vi "LcWebView_BubblePlot_Example.vi"() -> ()   [LabVIEW 2018, in "LcWebView.lvclass"]
doc: "Inject javascript arguments"
uses:
  LcWebView.lvclass
  plots/ctrls/PlotType.ctl
  plots/ctrls/GenericPlotOption.ctl
  plots/ctrls/LegendPosition.ctl
  C:/Users/ziggz/OneDrive/Documents/GitHub/LcWebView2/LcWebView/data/Microsoft.Web.WebView2.WinForms.dll
  Documents/GitHub/LcWebView2/LcWebView/data/Microsoft.Web.WebView2.WinForms.dll
panel:
  out "BrowserProcessId":u32
  out "Status Message":string
  in  "stop":bool
  in  "Web":refnum<k24>(container)
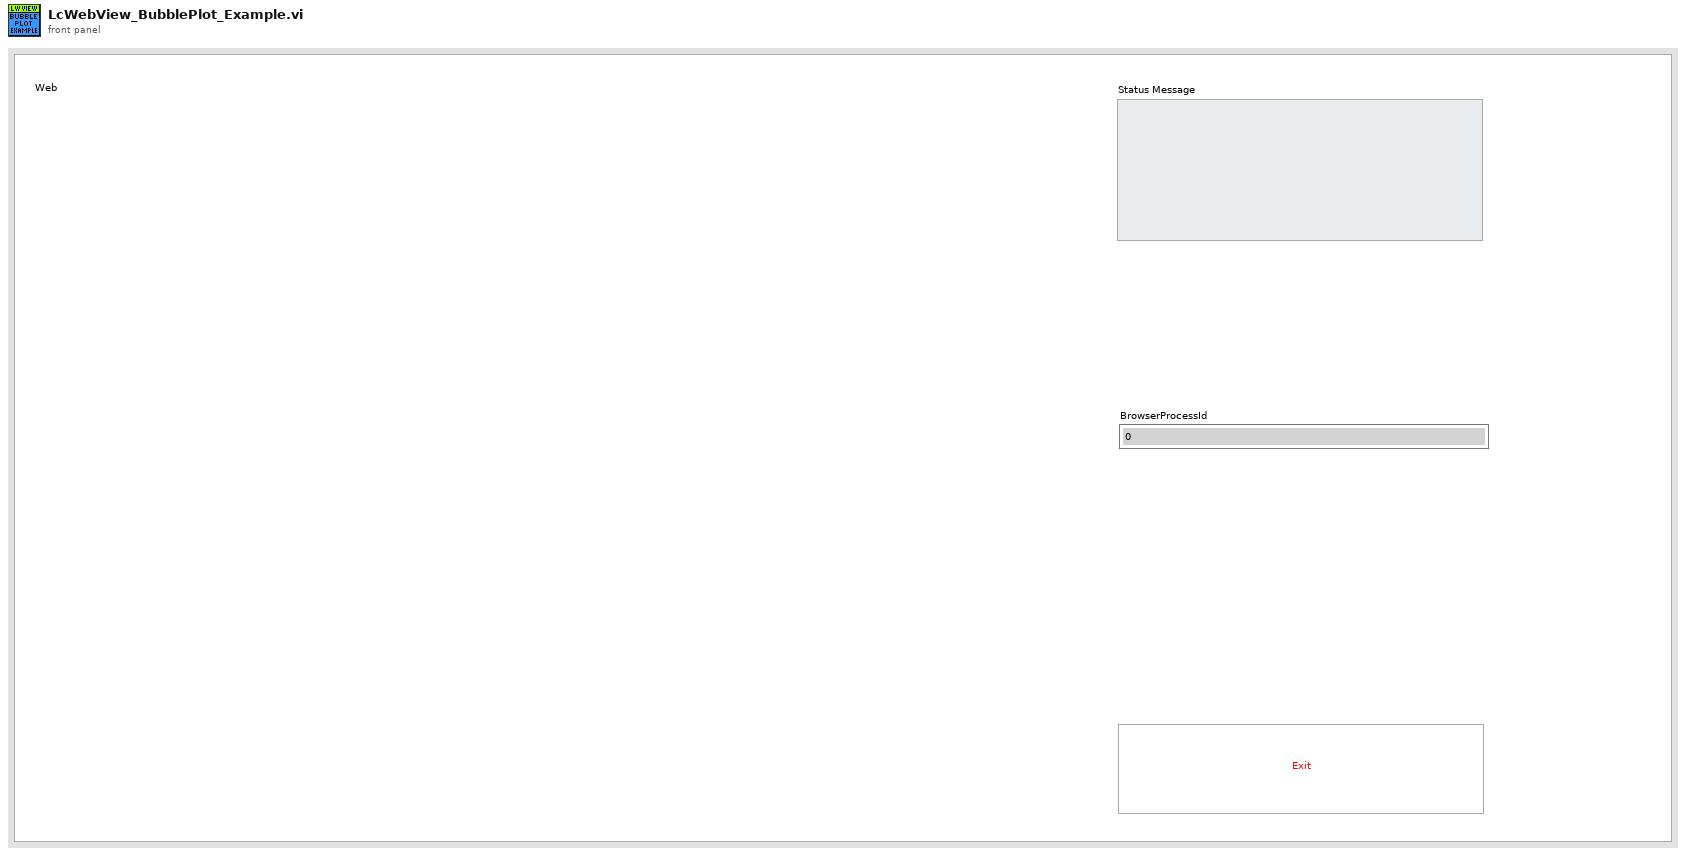
[diagram p1: front panel]
types:
  T1 = typedef "LcWebView.lvclass/GenericPlotOption.ctl" = cluster{"GraphTitle":string, "LegendDisplay":bool, "LegendPosition":T2}
  T2 = typedef "LcWebView.lvclass/LegendPosition.ctl" = enum16{"top", "right", "left", "bottom"}
  T3 = typedef "LcWebView.lvclass/PlotType.ctl" = enum16{"bar", "line", "pie", "doughnut", "scatter", "radar", "bubble", "polarArea"}
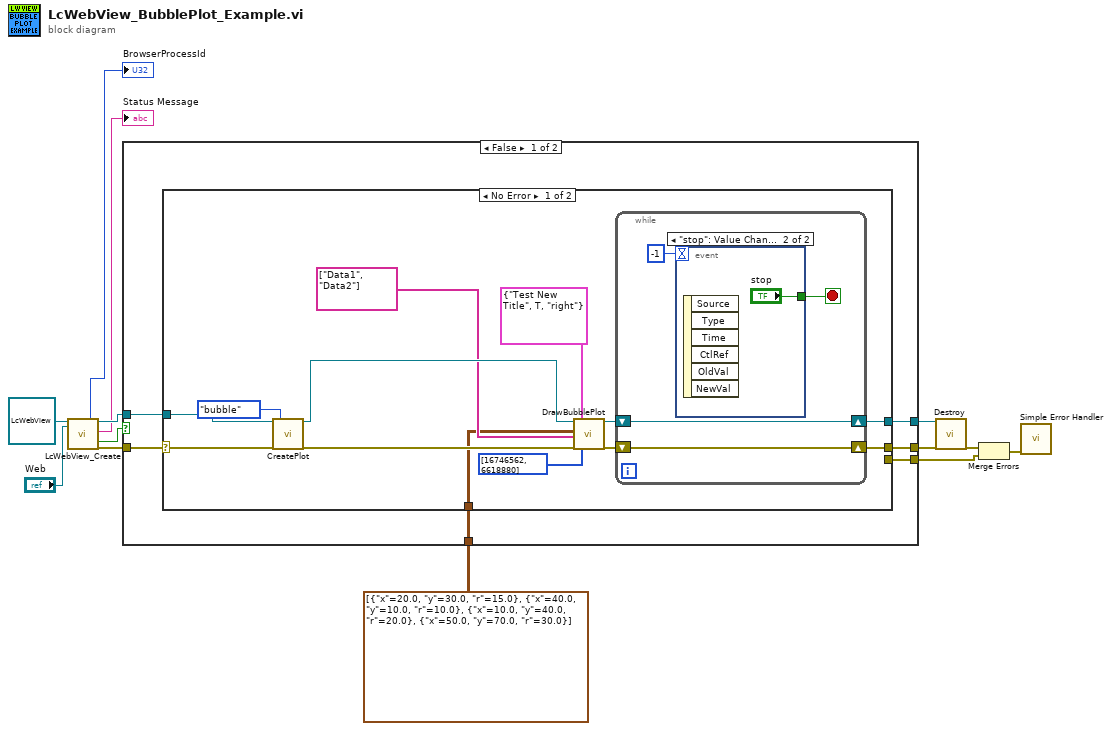
[diagram p0: block diagram]
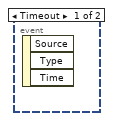
[diagram p2: hidden frame]
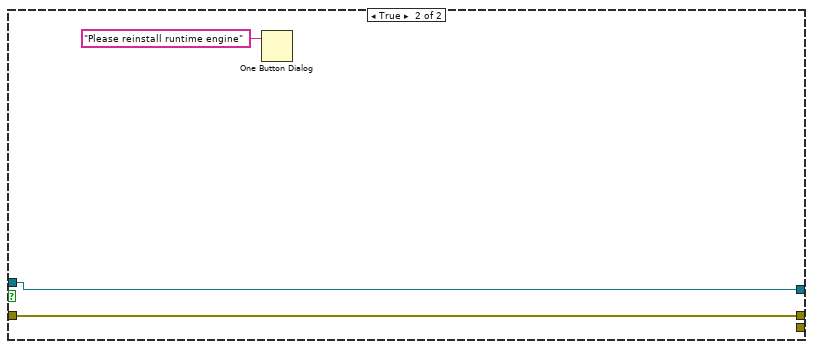
[diagram p4: hidden frame]
diagram:
  n1 = call "LcWebView_Create.vi"("reference in"=refnum<class "LcWebView.lvclass"> refnum, "Webview container"="Web") -> ("BrowserProcessId"=→"BrowserProcessId":u32, "reference out"=w11:refnum<class "LcWebView.lvclass">, "Status Message"=→"Status Message":string, "Reinstall Runtime"=w4:bool, "Error Out"=w10:errorcluster)  [unwired: 10 in, 3 out]
  n2 = case shown="False" w4 {
    tunnel: w11 -> [w19 w42]
    tunnel: w10 -> [w18 w41]
    tunnel: [w17 w42] -> w9
    tunnel: [w15 w41] -> w8
    tunnel: [w16 _] -> w5
    tunnel: cluster{"x":dbl, "y":dbl, "r":dbl}[][] [[{"x"=20.0, "y"=30.0, "r"=15.0}, {"x"=40.0, "y"=10.0, "r"=10.0}], [{"x"=10.0, "y"=40.0, "r"=20.0}, {"x"=50.0, "y"=70.0, "r"=30.0}]] ("BubblePlot.Dataset") -> [w14 _]
    frame False {
      n3 = case shown="No Error" w18 {
        selector: w18 -> [w30 w38]
        tunnel: w19 -> [w31 w39]
        tunnel: [w29 w39] -> w17
        tunnel: [w32 _] -> w15
        tunnel: [_ w38] -> w16
        tunnel: w14 -> [w20 _]
        frame No Error {
          n4 = call-dynamic "CreatePlot.vi"("reference in"=w31, "Error In"=w30, "PlotType"=PlotType."bubble") -> ("reference out"=w28:refnum<class "LcWebView.lvclass">, "Error Out"=w25:errorcluster)  [unwired: 15 in]
          n5 = call-dynamic "DrawBubblePlot.vi"("reference in"=w28, "BubblePlot.Dataset"=w20, "Scatter.DatasetLabels"=string[] ["Data1", "Data2"] ("DatasetLabels"), "Error In"=w25, "GenericPlotOptions"=T1 {"GraphTitle"="Test New Title", "LegendDisplay"=TRUE, "LegendPosition"=enum."right"}, "BubblePlot.PlotColours"=u32[] [16746562, 6618880] ("PlotColours")) -> ("reference out"=w27:refnum<class "LcWebView.lvclass">, "Error Out"=w26:errorcluster)  [unwired: 12 in]
          n6 = while {
            shift-right: [w36] -> w29
            shift-left: w27 -> [w36]
            shift-right: [w35] -> w32
            shift-left: w26 -> [w35]
            stop <- w33 stop-if-true
            n7 = event shown="[1] \"stop\": Value Change" {
              selector: _ -> [_ _]
              dyn-events: _ -> [_ _]
              timeout: -1 -> [_ _]
              tunnel: [_ "stop"] -> w33
              event Timeout {
                n8 = event-data() -> ()  [unwired: 1 in, 3 out]
              }
              event "stop": Value Change {
                n9 = event-data() -> ()  [unwired: 1 in, 6 out]
              }
            }
          }
        }
        frame Error {
        }
      }
    }
    frame True {
      n10 = One Button Dialog(message="Please reinstall runtime engine") -> ()  [unwired: 1 in, 1 out]
    }
  }
  n11 = call-dynamic "Destroy.vi"("reference in"=w9, "Error In"=w8) -> ("Error Out"=w7:errorcluster)  [unwired: 16 in, 1 out]
  n12 = Merge Errors(w7, w5) -> (w2:errorcluster)
  n13 = call <vilib>:"Simple Error Handler.vi"("error in (no error)"=w2) -> ()  [unwired: 4 in, 5 out]
